vi "RQST Comm Lookup Table_Actions.vi"(0 "ref in":T1, 5 "Connection In":T2, 7 "Index":i32, 9 "Method":T5, 11 "error in (no error)":errorcluster, 12 "Properties In":T4) -> (3 "All Properties":T4[](array[typedef]), 4 "reference out":T1, 6 "Connection Out":T2, 8 "All Connections":T2[](array[typedef]), 10 "Number of Connections":i32, 14 "Properties out":T4, 15 "error out":errorcluster {"code" min=0 max=0})   [LabVIEW 2015, in "J1939 Addon Engine.lvlib"]
uses:
  J1939 Addon Engine.lvlib
  Shared/Types/RQST Comm Lookup Table_Ref.ctl
  Shared/STM/Connection Manager/stm_ManagerStateVariables.ctl
  Shared/STM/TCP/stm_TCP Connection Info.ctl
  Shared/STM/_SubVIs/stm_MetaDataElement.ctl
  Shared/STM/Connection Manager/stm_TCPConnectionProperties.ctl
  Shared/STM/Connection Manager/stm_TCPConnectionMethod.ctl
  Shared/J1939 Addon Shared.lvlib
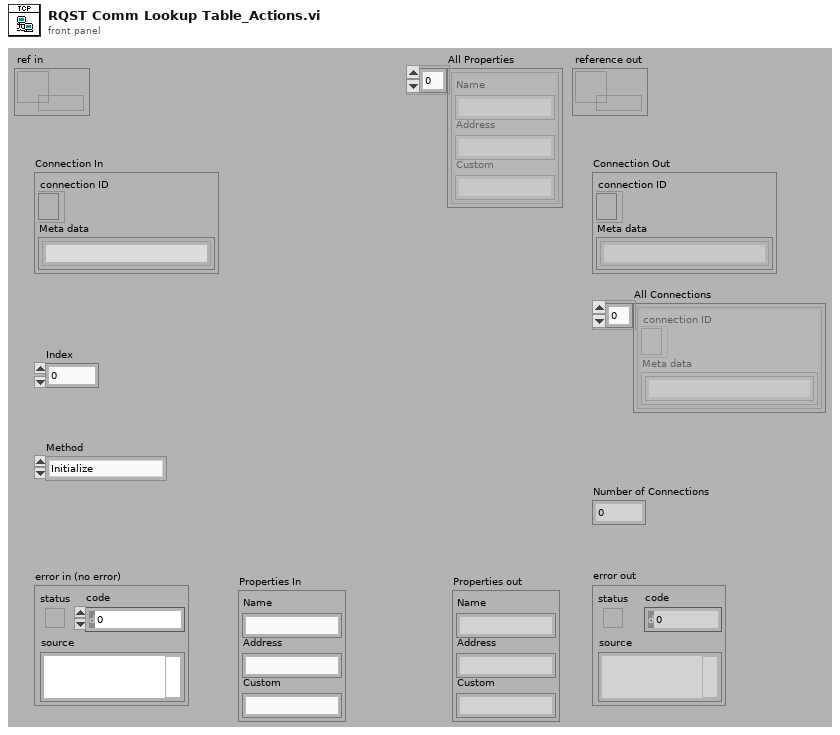
[diagram p1: front panel]
types:
  T1 = typedef "J1939 Addon Shared.lvlib/RQST Comm Lookup Table_Ref.ctl" = refnum<data-value>
  T2 = typedef "J1939 Addon Shared.lvlib/stm_TCP Connection Info.ctl" = cluster{"connection ID":refnum<k5>, "Meta data":T3[]}
  T3 = typedef "J1939 Addon Shared.lvlib/stm_MetaDataElement.ctl" = string
  T4 = typedef "J1939 Addon Shared.lvlib/stm_TCPConnectionProperties.ctl" = cluster{"Name":string, "Address":string, "Custom":string}
  T5 = typedef "J1939 Addon Shared.lvlib/stm_TCPConnectionMethod.ctl" = enum16{"Initialize", "Add Connection", "Set Properties", "Get Connection(s)", "Remove Connection", "Remove All Connections", "Get Connection Count"}
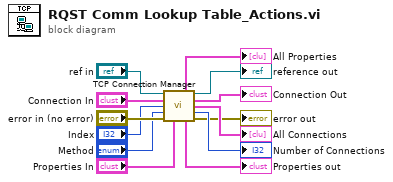
[diagram p0: block diagram]
diagram:
  n1 = call "TCP Connection Manager.vi"("TCP Ref"="ref in", "Connection In"="Connection In", "Index"="Index", "Method"="Method", "error in (no error)"="error in (no error)", "Properties In"="Properties In") -> ("All Properties"=→"All Properties":T4[], "TCP Ref out"=→"reference out":T1, "Connection Out"=→"Connection Out":T2, "All Connections"=→"All Connections":T2[], "Number of Connections"=→"Number of Connections":i32, "Properties out"=→"Properties out":T4, "error out"=→"error out":errorcluster)  [unwired: 3 in]
